vi "groundwater log header.vi"(5 "Worksheet Names":string[](array[string]), 7 "Groundwater Header":T1, 8 "error in (no error)":errorcluster, 11 "NI_report in":refnum<class "NI_report.lvclass">) -> (0 "error out":errorcluster, 3 "NI_report out":refnum<class "NI_report.lvclass">)   [LabVIEW 2016]
uses:
  <vilib>/Utility/NIReport.llb/NI_report.lvclass
  Groundwater header.ctl
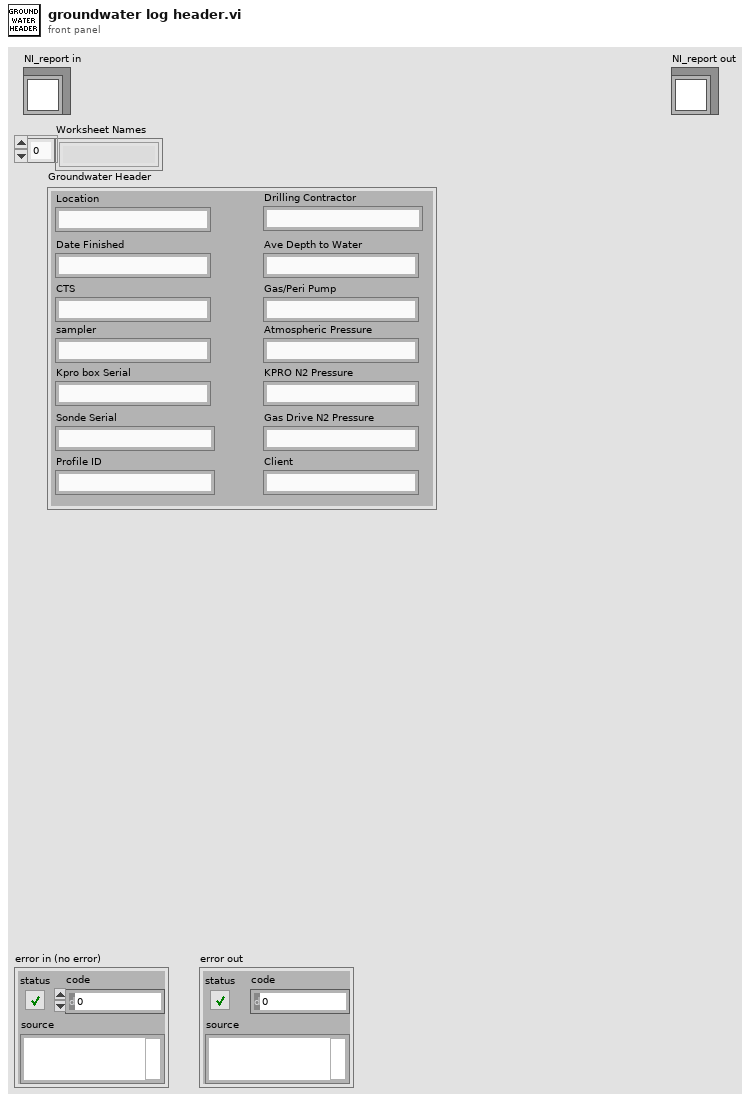
[diagram p1: front panel]
types:
  T1 = typedef "Groundwater header.ctl" = cluster{"Location":string, "Date Finished":string, "CTS":string, "sampler":string, "Kpro box Serial ":string, "Sonde Serial":string, "Drilling Contractor":string, "Ave Depth to Water":string, "Gas/Peri Pump":string, "Atmospheric Pressure":string, "KPRO N2 Pressure":string, "Gas Drive N2 Pressure":string, "Profile ID":string, "Client":string}
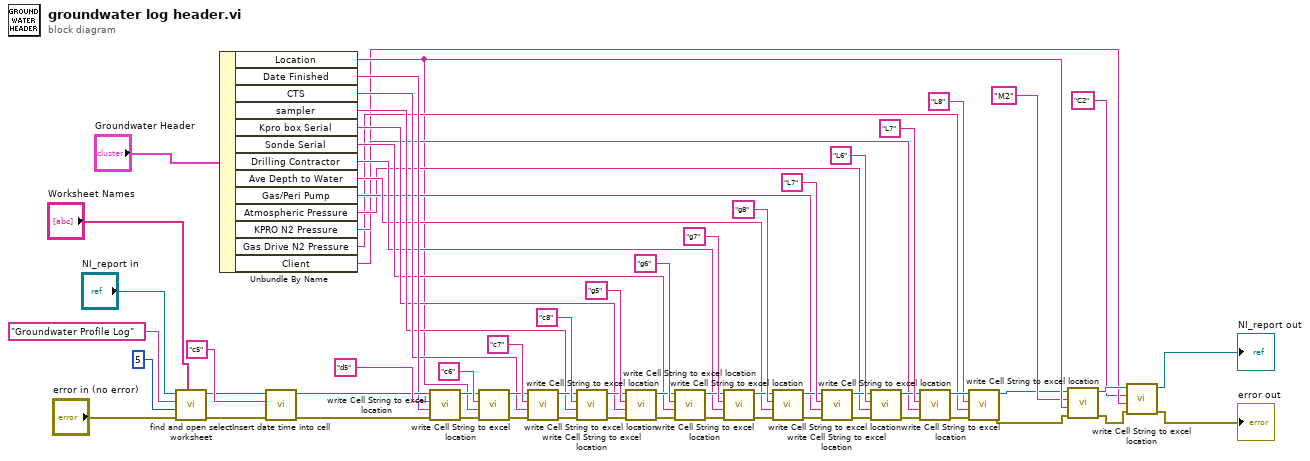
[diagram p0: block diagram]
diagram:
  n1 = call "find and open select worksheet.vi"("Worksheet Names"="Worksheet Names", "error in (no error)"="error in (no error)", "milliseconds to wait"=u32 5, "Worksheet Name in"="Groundwater Profile Log" ("Worksheet Name"), "NI_report in"="NI_report in") -> ("error out"=w28:errorcluster, "NI_report out"=w27:refnum<class "NI_report.lvclass">)  [unwired: 4 in, 1 out]
  n2 = Unbundle By Name("Groundwater Header") -> ("Location"=w10:string, "Date Finished"=w21:string, "CTS"=w20:string, "sampler"=w19:string, "Kpro box Serial"=w18:string, "Sonde Serial"=w17:string, "Drilling Contractor"=w16:string, "Ave Depth to Water"=w15:string, "Gas/Peri Pump"=w14:string, "Atmospheric Pressure"=w13:string, "KPRO N2 Pressure"=w12:string, "Gas Drive N2 Pressure"=w11:string, "Client"=w2:string)
  n3 = call "Insert date time into cell.vi"("error in (no error)"=w28, "Date/Time Cell"="c5", "NI_report in"=w27) -> ("error out"=w31:errorcluster, "NI_report out"=w30:refnum<class "NI_report.lvclass">)  [unwired: 7 in]
  n4 = call "write Cell String to excel location.vi"("error in (no error)"=w31, "input string"=w21, "cell's name"="d5", "NI_report in"=w30) -> ("error out"=w32:errorcluster, "NI_report out"=w33:refnum<class "NI_report.lvclass">)  [unwired: 6 in]
  n5 = call "write Cell String to excel location.vi"("error in (no error)"=w32, "input string"=w10, "cell's name"="c6", "NI_report in"=w33) -> ("error out"=w34:errorcluster, "NI_report out"=w35:refnum<class "NI_report.lvclass">)  [unwired: 6 in]
  n6 = call "write Cell String to excel location.vi"("error in (no error)"=w34, "input string"=w20, "cell's name"="c7", "NI_report in"=w35) -> ("error out"=w36:errorcluster, "NI_report out"=w37:refnum<class "NI_report.lvclass">)  [unwired: 6 in]
  n7 = call "write Cell String to excel location.vi"("error in (no error)"=w36, "input string"=w19, "cell's name"="c8", "NI_report in"=w37) -> ("error out"=w38:errorcluster, "NI_report out"=w40:refnum<class "NI_report.lvclass">)  [unwired: 6 in]
  n8 = call "write Cell String to excel location.vi"("error in (no error)"=w38, "input string"=w18, "cell's name"="g5", "NI_report in"=w40) -> ("error out"=w39:errorcluster, "NI_report out"=w41:refnum<class "NI_report.lvclass">)  [unwired: 6 in]
  n9 = call "write Cell String to excel location.vi"("error in (no error)"=w39, "input string"=w17, "cell's name"="g6", "NI_report in"=w41) -> ("error out"=w49:errorcluster, "NI_report out"=w50:refnum<class "NI_report.lvclass">)  [unwired: 6 in]
  n10 = call "write Cell String to excel location.vi"("error in (no error)"=w49, "input string"=w16, "cell's name"="g7", "NI_report in"=w50) -> ("error out"=w51:errorcluster, "NI_report out"=w52:refnum<class "NI_report.lvclass">)  [unwired: 6 in]
  n11 = call "write Cell String to excel location.vi"("error in (no error)"=w51, "input string"=w15, "cell's name"="g8", "NI_report in"=w52) -> ("error out"=w53:errorcluster, "NI_report out"=w54:refnum<class "NI_report.lvclass">)  [unwired: 6 in]
  n12 = call "write Cell String to excel location.vi"("error in (no error)"=w53, "input string"=w14, "cell's name"="L7", "NI_report in"=w54) -> ("error out"=w57:errorcluster, "NI_report out"=w58:refnum<class "NI_report.lvclass">)  [unwired: 6 in]
  n13 = call "write Cell String to excel location.vi"("error in (no error)"=w57, "input string"=w13, "cell's name"="L6", "NI_report in"=w58) -> ("error out"=w61:errorcluster, "NI_report out"=w62:refnum<class "NI_report.lvclass">)  [unwired: 6 in]
  n14 = call "write Cell String to excel location.vi"("error in (no error)"=w61, "input string"=w12, "cell's name"="L7", "NI_report in"=w62) -> ("error out"=w65:errorcluster, "NI_report out"=w66:refnum<class "NI_report.lvclass">)  [unwired: 6 in]
  n15 = call "write Cell String to excel location.vi"("error in (no error)"=w65, "input string"=w11, "cell's name"="L8", "NI_report in"=w66) -> ("error out"=w8:errorcluster, "NI_report out"=w7:refnum<class "NI_report.lvclass">)  [unwired: 6 in]
  n16 = call "write Cell String to excel location.vi"("error in (no error)"=w8, "input string"=w10, "cell's name"="M2", "NI_report in"=w7) -> ("error out"=w4:errorcluster, "NI_report out"=w6:refnum<class "NI_report.lvclass">)  [unwired: 6 in]
  n17 = call "write Cell String to excel location.vi"("error in (no error)"=w4, "input string"=w2, "cell's name"="C2", "NI_report in"=w6) -> ("error out"=→"error out":errorcluster, "NI_report out"=→"NI_report out":refnum<class "NI_report.lvclass">)  [unwired: 6 in]
